vi "Reset SmartMotor.vi"(0 "reference in":refnum<class "SmartMotor.lvclass">, 5 "error in (no error)":errorcluster) -> (14 "reference out":refnum<class "SmartMotor.lvclass">, 19 "error out":errorcluster)   [LabVIEW 2017, in "SmartMotor.lvclass"]
uses:
  SmartMotor.lvclass
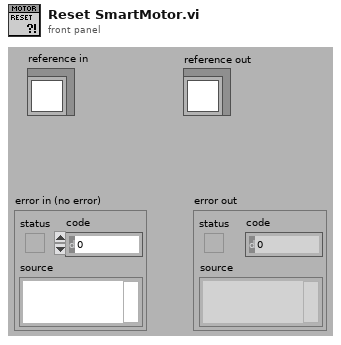
[diagram p1: front panel]
types:
  T1 = typedef "SmartMotor.lvclass/ObjectAttributes.ctl" = cluster{"SmartMotor Chain VISA Resource":refnum<visa-resource-name>, "SmartMotor Chain Address":i16, "Motor Absolute Position":i32, "Motor Relative Position":i32, "Motor Torque":i32, "Motor Voltage":i32, "Screwdriver Engaged":bool, "Screwdriver Torque Limit":i32, "Torque Monitor On/Off Status":bool, "Torque Monitor VI Reference":refnum<vi>, "Absolute Motor Torque (Filtered)":dbl, "SmartMotor Status":T2, "SmartMotor Error":T3}
  T2 = typedef "SmartMotor.lvclass/SmartMotor Status.ctl" = enum8{"Stopped", "Moving"}
  T3 = typedef "SmartMotor.lvclass/SmartMotor Error.ctl" = enum8{"None", "Read Error", "Low Voltage"}
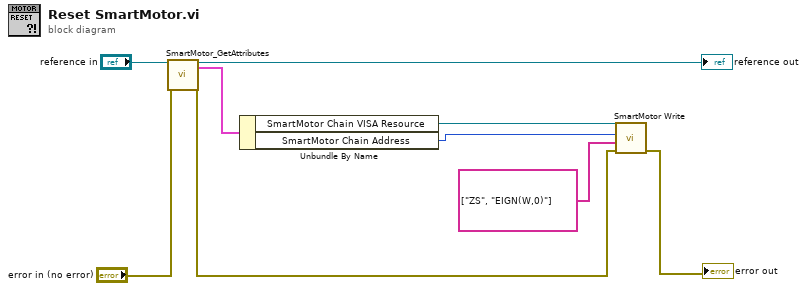
[diagram p0: block diagram]
diagram:
  n1 = call "SmartMotor_GetAttributes.vi"("reference in"="reference in", "error in (no error)"="error in (no error)") -> ("reference out"=→"reference out":refnum<class "SmartMotor.lvclass">, "Data"=w5:T1, "error out"=w1:errorcluster)  [unwired: 14 in, 1 out]
  n2 = Unbundle By Name(w5) -> ("SmartMotor Chain VISA Resource"=w3:refnum<visa-resource-name>, "SmartMotor Chain Address"=w2:i16)
  n3 = call "SmartMotor Write.vi"("VISA resource IN"=w3, "Motor Number"=w2, "Motor Command Array"=string[] ["ZS", "EIGN(W,0)"], "Error In"=w1) -> ("Error Out"=→"error out":errorcluster)  [unwired: 3 in, 2 out]
